vi "Calibration File Locate.vi"(11 "Base Path":path) -> (1 "SPL Calibration":path, 2 "Flow Calibration":path, 3 "Pressure Calibration":path)   [LabVIEW 2020, in "CollectionSupport.lvlib"]
uses:
  CollectionSupport.lvlib
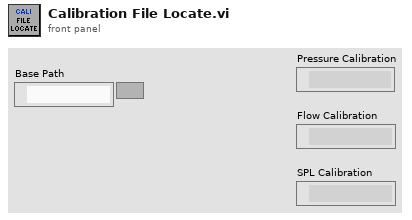
[diagram p1: front panel]
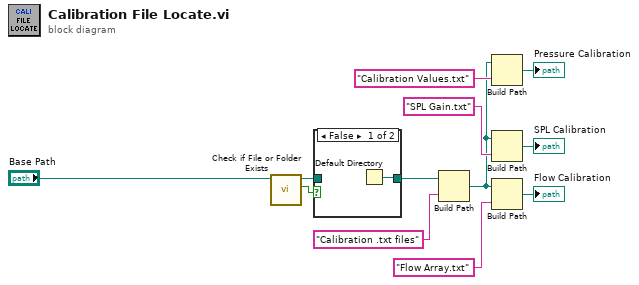
[diagram p0: block diagram]
diagram:
  n1 = call <vilib>:"Check if File or Folder Exists.vi"("path"="Base Path") -> ("file or folder exists?"=w3:bool, "dup path"=w2:path)  [unwired: 8 in, 1 out]
  n2 = case shown="False" w3 {
    tunnel: w2 -> [_ w14]
    tunnel: [w13 w14] -> w1
    frame False {
      n3 = Default Directory() -> (w13:path)
    }
    frame True {
    }
  }
  n4 = Build Path(base path=w1, name or relative path="Calibration .txt files") -> (appended path=w9:path)
  n5 = Build Path(base path=w9, name or relative path="Calibration Values.txt") -> (appended path=→"Pressure Calibration":path)
  n6 = Build Path(base path=w9, name or relative path="SPL Gain.txt") -> (appended path=→"SPL Calibration":path)
  n7 = Build Path(base path=w9, name or relative path="Flow Array.txt") -> (appended path=→"Flow Calibration":path)
